vi "login.vi"(1 "UserLibFile":path=path "D:/test.usr", 2 "Pwd":string, 3 "User":string caption="User Name:") -> (0 "Boolean":bool)   [LabVIEW 2020]
uses:
  <userlib>/_OpenG.lib/md5/md5.llb/MD5 Message Digest (Hexadecimal String)__ogtk.vi
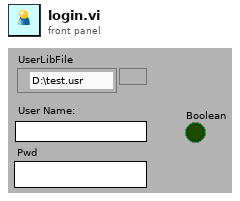
[diagram p1: front panel]
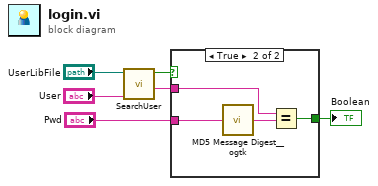
[diagram p0: block diagram]
diagram:
  n1 = call "SearchUser.vi"("User"="User", "UserLibFile"="UserLibFile") -> ("Pwd"=w2:string, "Exist?"=w4:bool)  [unwired: 6 in, 2 out]
  n2 = case shown="True" w4 {
    selector: w4 -> [w7 _]
    tunnel: "Pwd" -> [_ w11]
    tunnel: w2 -> [_ w9]
    tunnel: [w7 w8] -> w1
    frame False {
    }
    frame True {
      n3 = call-poly <userlib>:"MD5 Message Digest__ogtk.vi"("Message"=w11) -> ("MD5 Message Digest"=w10:string)
      n4 = Equal?(x=w9, y=w10) -> (x = y?=w8:bool)
    }
  }
  "Boolean" <- w1
